vi "Template - Scope Acquire Waveform.vi"() -> ()   [LabVIEW 2020]
doc: "This example shows how to use autosetup and acquire a waveform on a single channel."
uses:
  <instrlib>/_Template - Scope/Public/Data/Read Waveform (Single).vi
  <instrlib>/_Template - Scope/Template - Scope.lvlib
panel:
  in  "Maximum Time (10000 ms)":u32=10000
  in  "Serial Configuration":T1={"Baud Rate"=9600, "Parity"=0, "Data Bits"=7, "Stop Bits"=10, "Flow Control"=0} {"Flow Control" items=["None", "XON/XOFF", "RTS/CTS", "XON/XOFF & RTS/CTS", "DTR/DSR", "XON/XOFF & DTR/DSR"]; "Stop Bits" items=["1.0"=10, "1.5"=15, "2.0"=20]; "Data Bits" items=["7"=7, "8"=8]; "Parity" items=["None", "Odd", "Even", "Mark", "Space"]; "Baud Rate" items=["300"=300, "600"=600, "1200"=1200, "2400"=2400, "4800"=4800, "9600"=9600, "19200"=19200]}
  in  "Probe Attenuation (10.0)":dbl=10.0
  out "Waveform Data":waveform(dbl)(graph)
  in  "Channel (1: Channel 1)":u16(ring)=1 items=["Channel 1"=1, "Channel 2"=2]
  in  "VISA resource name":refnum<visa-resource-name>
  # "(c) 2014 <Enter Company Name Here>.  ALL RIGHTS RESERVED."
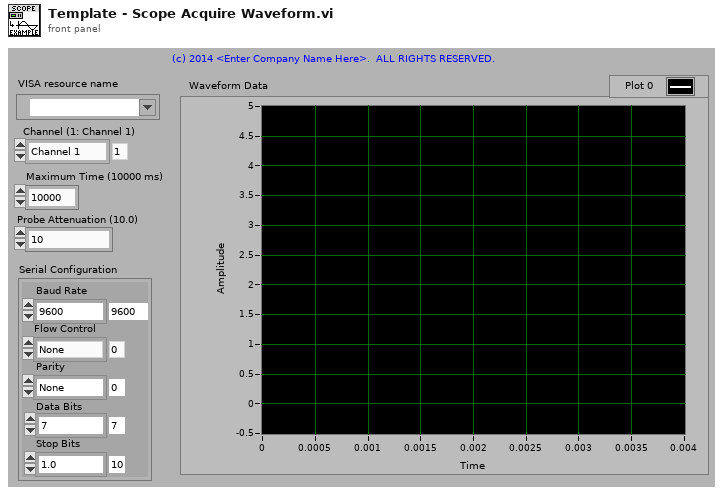
[diagram p1: front panel]
types:
  T1 = cluster{"Baud Rate":u32, "Parity":u16, "Data Bits":u16, "Stop Bits":u16, "Flow Control":u16}
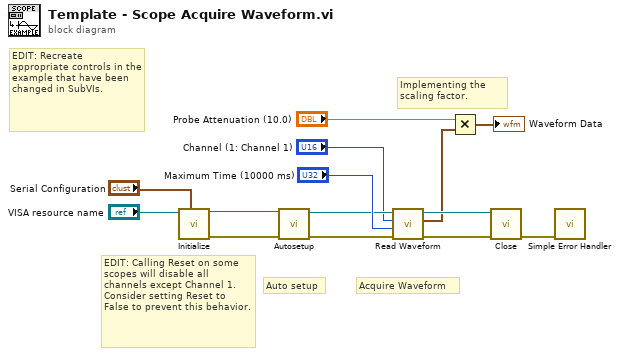
[diagram p0: block diagram]
diagram:
  # "EDIT: Calling Reset on some scopes will disable all channels except Channel 1. Consider setting Reset to False to prevent this behavior."
  # "EDIT: Recreate appropriate controls in the example that have been changed in SubVIs."
  # "Implementing the scaling factor."
  # "Acquire Waveform"
  # "Auto setup"
  n1 = call <instrlib>:"Initialize.vi"("Serial Configuration"="Serial Configuration", "VISA resource name"="VISA resource name") -> ("error out"=w12:errorcluster, "VISA resource name out"=w11:refnum<visa-resource-name>)  [unwired: 8 in]
  n2 = call <instrlib>:"Autosetup.vi"("error in (no error)"=w12, "VISA resource name"=w11) -> ("error out"=w1:errorcluster, "VISA resource name out"=w3:refnum<visa-resource-name>)  [unwired: 8 in]
  n3 = call-poly <instrlib>:"Read Waveform.vi"("error in (no error)"=w1, "Maximum Time (10000 ms)"="Maximum Time (10000 ms)", "Channel (1: Channel 1)"="Channel (1: Channel 1)", "VISA resource name"=w3) -> ("error out"=w5:errorcluster, "Waveform Data"=w6:waveform(dbl), "VISA resource name out"=w7:refnum<visa-resource-name>)  [unwired: 5 in]
  n4 = Multiply(x="Probe Attenuation (10.0)", y=w6) -> (x*y=→"Waveform Data":waveform(dbl))
  n5 = call <instrlib>:"Close.vi"("error in (no error)"=w5, "VISA resource name"=w7) -> ("error out"=w14:errorcluster)  [unwired: 9 in]
  n6 = call <vilib>:"Simple Error Handler.vi"("error in (no error)"=w14) -> ()  [unwired: 4 in, 5 out]
